vi "RichToFlatcif_management_common_PluginMetadata.vi"(5 "OutputClusterType":T1, 11 "InputCluster":T2) -> (3 "OutputCluster":T1)   [LabVIEW 2021, in "CIFCorePlugin_server.lvlib"]
uses:
  CIFCorePlugin_server.lvlib
  cif_management_common_PluginMetadata.ctl
  cif_management_common_PluginMetadata_Flat.ctl
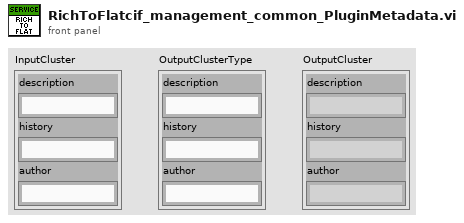
[diagram p1: front panel]
types:
  T1 = typedef "CIFCorePlugin_server.lvlib/cif_management_common_PluginMetadata_Flat.ctl" = cluster{"description":string, "history":string, "author":string}
  T2 = typedef "CIFCorePlugin_server.lvlib/cif_management_common_PluginMetadata.ctl" = cluster{"description":string, "history":string, "author":string}
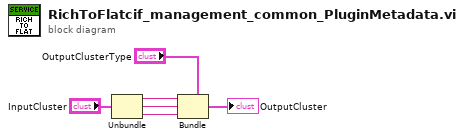
[diagram p0: block diagram]
diagram:
  n1 = Unbundle "Unbundle"("InputCluster") -> ("description"=w3:string, "history"=w2:string, "author"=w1:string)
  n2 = Bundle "Bundle"(cluster="OutputClusterType", "description"=w3, "history"=w2, "author"=w1) -> (→"OutputCluster":T1)
